vi "Do.vi"(8 "error in (no error)":errorcluster, 10 "Actor in":refnum<class "Actor.lvclass">, 11 "Conceret Initialize Edit Test Channel Msg in":refnum<class "Conceret Initialize Edit Test Channel Msg.lvclass">) -> (0 "error out":errorcluster, 2 "Actor out":refnum<class "Actor.lvclass">)   [LabVIEW 2013, in "Edit Test Channel View.lvlib" / "Conceret Initialize Edit Test Channel Msg.lvclass"]
doc: "(<B>Filename</B>: Actor Framework.lvlib:Message.lvclass:Do.vi)\n\nDefines what a message does when it is received by an actor. Generally, a message instructs an actor to invoke one of its methods.\n\nBy default, this method does nothing. A child class must override it to define behavior. Create a child class by using the Actor Framework Message Maker dialog box."
uses:
  Conceret Initialize Edit Test Channel Msg.lvclass
  <vilib>/ActorFramework/Actor/Actor.lvclass
  Edit Test Channel View/Edit Test Channel View.lvclass
  Models/Edit Test Channel Model Messages/Abstract Initialize Edit Test Channel Msg/Abstract Initialize Edit Test Channel Msg.lvclass
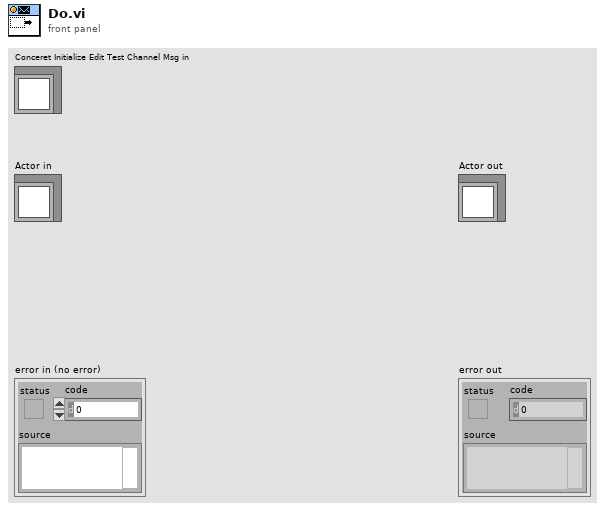
[diagram p1: front panel]
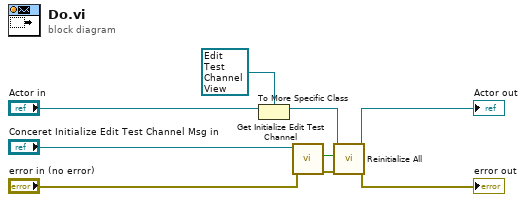
[diagram p0: block diagram]
diagram:
  n1 = To More Specific Class(target class=refnum<class "Edit Test Channel View.lvclass"> refnum ("Edit Test Channel View.lvlib:Edit Test Channel View.lvclass"), reference="Actor in") -> (specific class reference=w6:refnum<class "Edit Test Channel View.lvclass">)  [unwired: 1 in, 1 out]
  n2 = call "Get Initialize Edit Test Channel.vi"("error in (no error)"="error in (no error)", "Abstract Initialize Edit Test Channel Msg in"="Conceret Initialize Edit Test Channel Msg in") -> ("error out"=w5:errorcluster, "Initialize Edit Test Channel"=w1:bool)  [unwired: 7 in, 1 out]
  n3 = call "Reinitialize All.vi"("error in (no error)"=w5, "Initialize Edit Test Channel"=w1, "Create Test Channel View in"=w6) -> ("error out"=→"error out":errorcluster, "Create Test Channel View out"=→"Actor out":refnum<class "Edit Test Channel View.lvclass">)  [unwired: 7 in]
